vi "Modify SysDef.vi"(5 "Description":string, 7 "Creator":string, 8 "error in (no error)":errorcluster, 9 "IP":string, 10 "Name":string, 11 "Project Root Path":path) -> (0 "error out":errorcluster, 2 "Name dup":string, 3 "Project Root Path dup":path)   [LabVIEW 2013, in "Project Wizard.lvlib"]
uses:
  Project Wizard.lvlib
  NationalInstruments.VeriStand.SystemDefinitionAPI
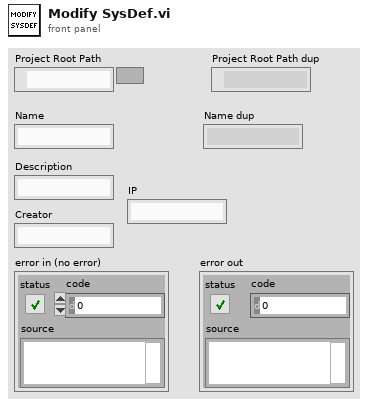
[diagram p1: front panel]
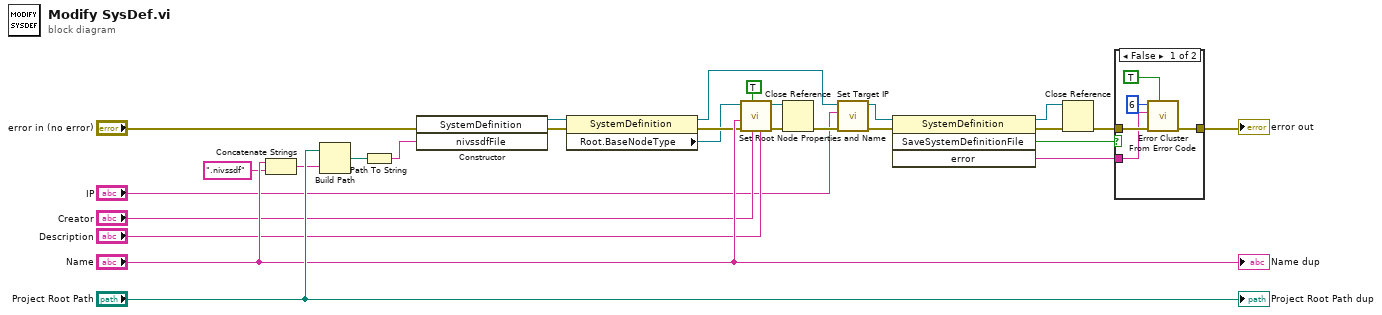
[diagram p0: block diagram]
diagram:
  n1 = Concatenate Strings("Name", ".nivssdf" ("string")) -> (w21:string)
  n2 = Build Path(base path="Project Root Path", name or relative path=w21) -> (appended path=w23:path)
  n3 = Path To String(path=w23) -> (string=w19:string)
  n4 = constructor class="SystemDefinition"(error in="error in (no error)", "nivssdfFile"=w19) -> (reference out=w8:refnum<k24>, error out=w22:errorcluster)  [unwired: 2 in, 2 out]
  n5 = property class="SystemDefinition"(reference=w8, error in=w22) -> (reference out=w2:refnum<k24>, error out=w18:errorcluster, "Root.BaseNodeType"=w7:refnum<k24>)
  n6 = call "Set Root Node Properties and Name.vi"("Description"="Description", "Creator"="Creator", "Skip search (F)"=TRUE, "error in (no error)"=w18, "Name"="Name", "Doc in"=w7) -> ("error out"=w10:errorcluster, "Doc out"=w9:refnum<k24>)  [unwired: 4 in]
  n7 = Close Reference(reference=w9, error in (no error)=w10) -> (error out=w17:errorcluster)
  n8 = call "Set Target IP.vi"("error in (no error)"=w17, "IP"="IP", "system definition in"=w2) -> ("error out"=w4:errorcluster, "system definition out"=w3:refnum<k24>)  [unwired: 7 in]
  n9 = invoke class="SystemDefinition" method="SaveSystemDefinitionFile"(reference=w3, error in=w4) -> (reference out=w15:refnum<k24>, error out=w16:errorcluster, "SaveSystemDefinitionFile"=w13:bool, "error"=w12:string)  [unwired: 2 in]
  n10 = Close Reference(reference=w15, error in (no error)=w16) -> (error out=w14:errorcluster)
  n11 = case shown="False" w13 {
    tunnel: w14 -> [w32 w33]
    tunnel: w12 -> [w31 _]
    tunnel: [w28 w33] -> w27
    frame False {
      n12 = call <vilib>:"Error Cluster From Error Code.vi"("show call chain? (False)"=TRUE, "error in (no error)"=w32, "error message (\"\")"=w31, "error code (0)"=6) -> ("error out"=w28:errorcluster)  [unwired: 5 in]
    }
    frame True {
    }
  }
  "error out" <- w27
  "Project Root Path dup" <- "Project Root Path"
  "Name dup" <- "Name"
